vi "TellParent.vi"(6 "Error":errorcluster, 10 "Msg":T1 {"Metadata"."AbsoluteTime" format="%<%x %.3X>T"}, 11 "Actor":refnum<class "Actor.lvclass">) -> (3 "Actor":refnum<class "Actor.lvclass">, 4 "Error":errorcluster)   [LabVIEW 2020, in "_Template.lvlib" / "{{Msg}}.lvlib"]
uses:
  {{Msg}}.lvlib
  Msg/Msg.lvclass
  jettl/jettl/jettl.lvlib
  jettl/jettl/Actor/Actor.lvclass
  jettl/jettl/Lifecycle.ctl
  jettl/jettl/Metadata.ctl
  Msg.ctl
  jettl/jettl/Metadata/Metadata.lvclass
  jettl/jettl/Origin.ctl
panel:
  # "This front panel should not be manipulated."
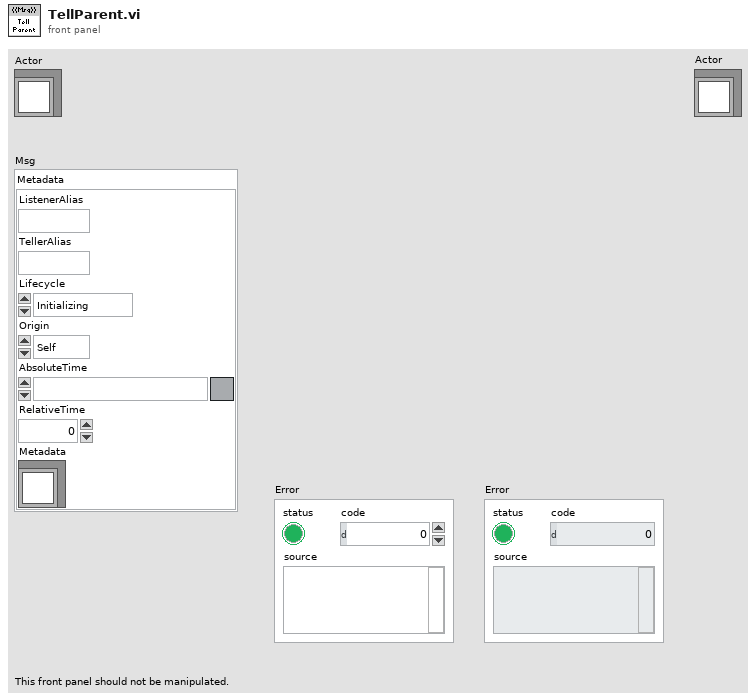
[diagram p1: front panel]
types:
  T1 = typedef "_Template.lvlib/{{Msg}}.lvlib/Msg.ctl" = cluster{"Metadata":T2}
  T2 = typedef "jettl.lvlib/Metadata.ctl" = cluster{"ListenerAlias":string, "TellerAlias":string, "Lifecycle":T3, "Origin":T4, "AbsoluteTime":timestamp, "RelativeTime":dbl, "Metadata":refnum<class "Metadata.lvclass">}
  T3 = typedef "jettl.lvlib/Lifecycle.ctl" = enum16{"Initializing", "SettingUp", "Starting", "Running", "Stopping", "TearingDown", "Terminated"}
  T4 = typedef "jettl.lvlib/Origin.ctl" = enum16{"Self", "Parent", "Child"}
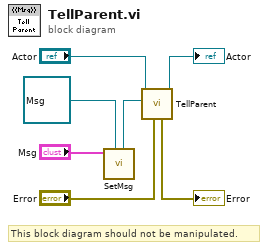
[diagram p0: block diagram]
diagram:
  # "This block diagram should not be manipulated."
  n1 = call "SetMsg.vi"("Message"=refnum<class "Msg.lvclass"> refnum ("_Template.lvlib:MessageTemplate.lvlib:{{Name}}.lvlib:ConcreteMessage.lvclass"), "PayloadCluster"="Msg") -> ("Message"=w4:refnum<class "Msg.lvclass">)  [unwired: 9 in]
  n2 = call "TellParent.vi"("Error"="Error", "Message"=w4, "Actor"="Actor") -> ("Actor"=→"Actor":refnum<class "Actor.lvclass">, "Error"=→"Error":errorcluster)  [unwired: 7 in]
